vi "tatrocki_10_sub_2.vi"(8 "error in (no error)":errorcluster) -> (3 "Boolean":bool)   [LabVIEW 2020]
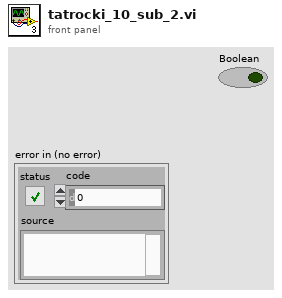
[diagram p1: front panel]
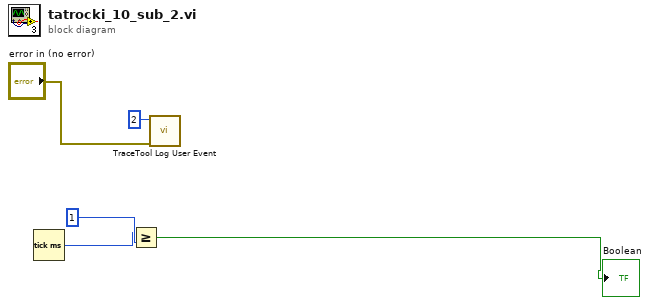
[diagram p0: block diagram]
diagram:
  n1 = Tick Count (ms)() -> (millisecond timer value=w2:u32)
  n2 = Greater Or Equal?(x=w2, y=u32 1 ("x")) -> (x >= y?=→"Boolean":bool)
  n3 = call <vilib>:"TraceTool Log User Event.vi"("error in (no error)"="error in (no error)", "Event ID (0-255)"=u32 2) -> ()  [unwired: 9 in, 1 out]
